vi "Stop.vi"(8 "error in (no error)":errorcluster, 11 "Electrophysiology in":refnum<class "Electrophysiology.lvclass">) -> (0 "error out":errorcluster, 3 "Electrophysiology out":refnum<class "Electrophysiology.lvclass">)   [LabVIEW 2010, in "Electrophysiology.lvclass"]
uses:
  Electrophysiology.lvclass
  AcquireTraces/AcquireTraces.lvclass
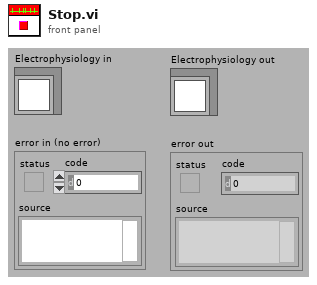
[diagram p1: front panel]
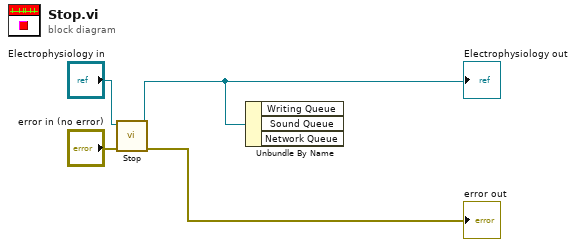
[diagram p0: block diagram]
diagram:
  n1 = call-parent "Stop.vi"("error in (no error)"="error in (no error)", "Electrophysiology in"="Electrophysiology in") -> ("error out"=→"error out":errorcluster, "Electrophysiology out"=w1:refnum<class "Electrophysiology.lvclass">)  [unwired: 8 in]
  "Electrophysiology out" <- w1
  n2 = Unbundle By Name(w1) -> ()  [unwired: 3 out]
